vi "Get Software Details extended (Array).vi"(8 "error in (no error)":errorcluster, 10 "Number of Elements":i32, 11 "Enumerator in":u64) -> (0 "error out":errorcluster, 3 "Software Components":T1[](array[typedef]) {"Visibility Type" items=["standard", "hidden", "system", "unknown", "startup", "image", "essential"]})   [LabVIEW 2020, in "nisyscfg.lvlib"]
uses:
  <vilib>/nisyscfg/nisyscfg.lvlib
  <vilib>/nisyscfg/Software Extended.ctl
  <vilib>/nisyscfg/Component Type.ctl
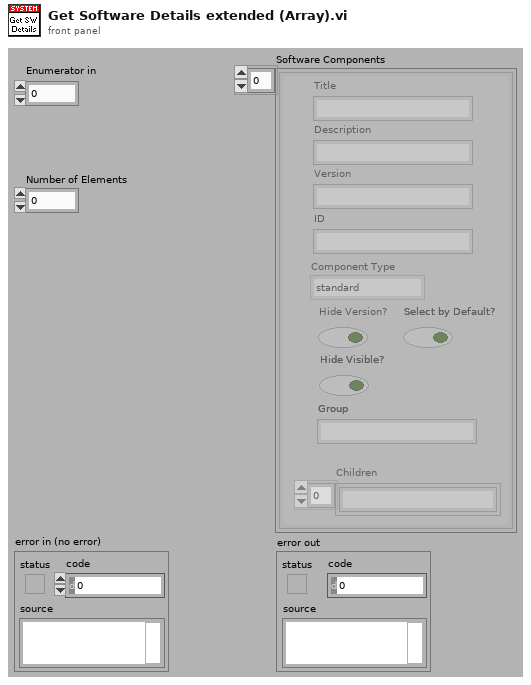
[diagram p1: front panel]
types:
  T1 = typedef "nisyscfg.lvlib/Software Extended.ctl" = cluster{"Description":string, "ID":string, "Version":string, "Title":string, "Visibility Type":T2, "Hide Version?":bool, "Children":string[], "Select by Default?":bool, "Hide Visible?":bool, "Group":string}
  T2 = typedef "nisyscfg.lvlib/Component Type.ctl" = u32
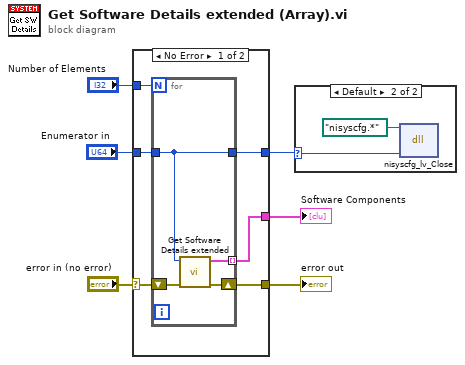
[diagram p0: block diagram]
diagram:
  n1 = case shown="No Error" "error in (no error)" {
    selector: "error in (no error)" -> [w12 w18]
    tunnel: [w11 w18] -> w5
    tunnel: "Enumerator in" -> [w10 w17]
    tunnel: [w9 _] -> w3
    tunnel: "Number of Elements" -> [w8 _]
    tunnel: [w7 w17] -> w1
    frame No Error {
      n2 = for {
        N: w8 -> [_]
        shift-right: [w15] -> w11
        shift-left: w12 -> [w16]
        tunnel: w10 -> [w13]
        tunnel: [w14] -> w9 mode=indexing
        tunnel: [w13] -> w7
        n3 = call <vilib>:"Get Software Details extended.vi"("error in (no error)"=w16, "Software Item"=w13) -> ("error out"=w15:errorcluster, "Software Extended Info"=w14:T1)  [unwired: 8 in]
      }
    }
    frame Error {
    }
  }
  "error out" <- w5
  "Software Components" <- w3
  n4 = case shown="Default" w1 {
    selector: w1 -> [_ w19]
    frame 0 {
      # "No need to call Close\non an empty enum."
    }
    frame Default {
      n5 = dll-call lib="nisyscfg.*" fn="nisyscfg_lv_Close" label="Close"(path in=path "nisyscfg.*", "expertsEnum"=w19) -> ()  [unwired: 3 in, 3 out]
    }
  }
